vi "Assign Pixel to Wing Sector (FPGA).vi"(6 "Pixel Intensity In":u8, 7 "Right Wing?":bool, 8 "Sector Parameters":T1, 9 "Pixel Y":u16, 10 "Pixel X":u16) -> (1 "Pixel Intensity Out":u8, 2 "sector #":u8, 3 "output valid":bool)   [LabVIEW 2013, in "FPGA Image Processing.lvlib"]
uses:
  FPGA Image Processing.lvlib
  Sector/Accumulate/Sector Parameter Cluster.ctl
  <vilib>/rvi/FXPMathLib/FxpRectToPolar/subVIs/nifxpmath_RectToPolar_SimConfig.ctl
  <vilib>/rvi/FXPMathLib/FxpDiv/subVIs/nifxpmath_Div_SimConfig.ctl
  <vilib>/rvi/FXPMathLib/FxpRectToPolar/simVIs/DllFxpRectToPolarTemp_sub.vi
  <vilib>/rvi/FXPMathLib/FxpDiv/simVIs/DllFxpDivTemp_sub.vi
  <vilib>/rvi/FXPMathLib/FxpSub/XNode/nifxpmath_Sub.xnode
  <vilib>/rvi/FXPMathLib/FxpRectToPolar/XNode/nifxpmath_RectToPolar.xnode
  <vilib>/rvi/FXPMathLib/FxpAdd/XNode/nifxpmath_Add.xnode
  <vilib>/rvi/FXPMathLib/FxpDiv/XNode/nifxpmath_Div.xnode
  <vilib>/rvi/FXPMathLib/sim/FxpSim.dll
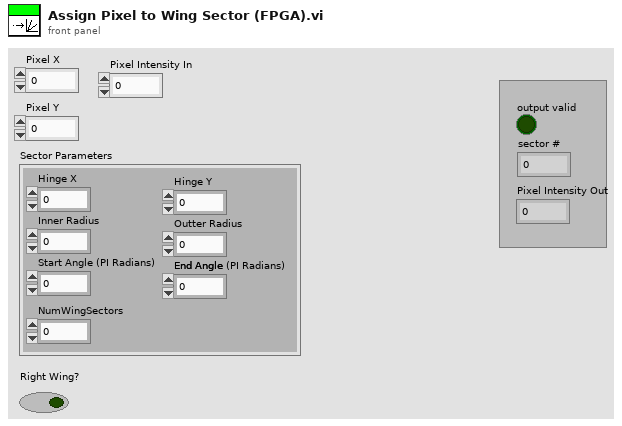
[diagram p1: front panel]
types:
  T1 = typedef "Sector Parameter Cluster.ctl" = cluster{"Start Angle":fxp<+,17,3>, "End Angle":fxp<+,17,3>, "Inner Radius":u16, "Outter Radius":u16, "Hinge X":u16, "Hinge Y":u16, "NumWingSectors":u8}
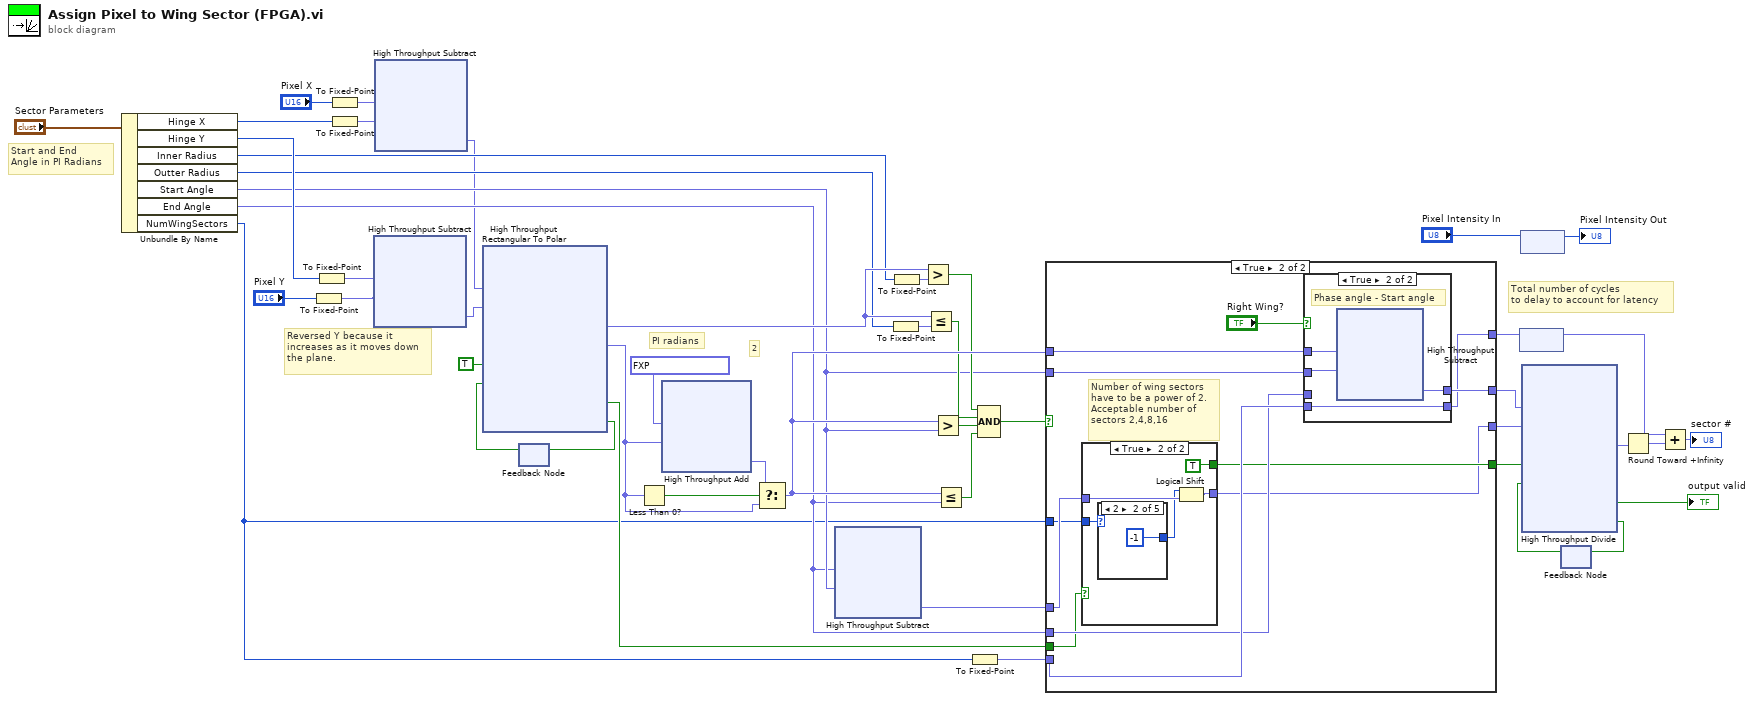
[diagram p0: block diagram]
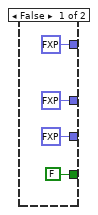
[diagram p2: hidden frame]
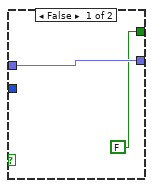
[diagram p3: hidden frame]
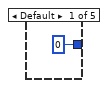
[diagram p4: hidden frame]
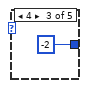
[diagram p5: hidden frame]
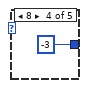
[diagram p6: hidden frame]
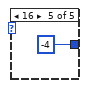
[diagram p7: hidden frame]
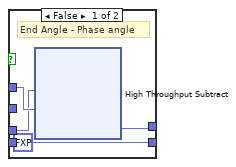
[diagram p8: hidden frame]
diagram:
  # "Reversed Y because it\nincreases as it moves down\nthe plane."
  # "PI radians"
  # "Total number of cycles\nto delay to account for latency"
  # "Start and End\nAngle in PI Radians"
  # "2"
  n1 = Unbundle By Name("Sector Parameters") -> ("Hinge X"=w29:u16, "Hinge Y"=w28:u16, "Inner Radius"=w27:u16, "Outter Radius"=w26:u16, "Start Angle"=w25:fxp<+,17,3>, "End Angle"=w24:fxp<+,17,3>, "NumWingSectors"=w3:u8)
  n2 = To Fixed-Point(number="Pixel Y") -> (fixed-point=w8:fxp<+,11,11>)  [unwired: 1 in]
  n3 = To Fixed-Point(number=w28) -> (fixed-point=w9:fxp<+,11,11>)  [unwired: 1 in]
  n4 = To Fixed-Point(number="Pixel X") -> (fixed-point=w7:fxp<+,11,11>)  [unwired: 1 in]
  n5 = To Fixed-Point(number=w29) -> (fixed-point=w6:fxp<+,11,11>)  [unwired: 1 in]
  n6 = xnode "High Throughput Subtract"("x"=w9, "y"=w8) -> ("x-y"=w22:fxp<+/-,12,12>)
  n7 = xnode "High Throughput Subtract"("x"=w7, "y"=w6) -> ("x-y"=w21:fxp<+/-,12,12>)
  n8 = feedback #1() -> (w37:bool)  [unwired: 1 in]
  n9 = xnode "High Throughput Rectangular To Polar"("x"=w21, "y"=w22, "input valid"=TRUE, "ready for output (T)"=w37) -> ("magnitude"=w47:fxp<+,12,12>, "phase (pi)"=w43:fxp<+/-,16,2>, "output valid"=w4:bool, "ready for input"=w38:bool)
  n10 = feedback-in #1(w38) -> ()
  n11 = Less Than 0?(x=w43) -> (x < 0?=w44:bool)
  n12 = xnode ("High Throughput Add")("x"=fxp<+/-,16,2> 1.99993896484375 ("y"), "y"=w43) -> ("x+y"=w42:fxp<+/-,17,3>)
  n13 = Select(t=w42, s=w44, f=w43) -> (s? t:f=w40:fxp<+/-,17,3>)
  n14 = xnode ("High Throughput Subtract")("x"=w24, "y"=w25) -> ("x-y"=w5:fxp<+/-,17,6>)
  n15 = To Fixed-Point(number=w26) -> (fixed-point=w46:fxp<+,16,16>)  [unwired: 1 in]
  n16 = To Fixed-Point(number=w27) -> (fixed-point=w48:fxp<+,16,16>)  [unwired: 1 in]
  n17 = Greater?(x=w47, y=w48) -> (0:w34:bool)
  n18 = Less Or Equal?(x=w47, y=w46) -> (x <= y?=w33:bool)
  n19 = Greater?(x=w40, y=w25) -> (0:w32:bool)
  n20 = Less Or Equal?(x=w40, y=w24) -> (x <= y?=w31:bool)
  n21 = To Fixed-Point(number=w3) -> (fixed-point=w23:fxp<+,8,8>)  [unwired: 1 in]
  n22 = Compound Arithmetic op=AND(w34, w33, w32, w31) -> (w45:bool)
  n23 = case shown="True" w45 {
    tunnel: w40 -> [_ w64]
    tunnel: w25 -> [_ w63]
    tunnel: [fxp<+/-,17,6> 0.0 ("x-y") w53] -> w16
    tunnel: w24 -> [_ w60]
    tunnel: w23 -> [_ w61]
    tunnel: [fxp<+/-,19,5> 0.0 ("x-y") w59] -> w17
    tunnel: [FALSE ("output valid") w54] -> w15
    tunnel: [fxp<+,8,8> 0.0 w58] -> w12
    tunnel: w5 -> [_ w57]
    tunnel: w4 -> [_ w56]
    tunnel: w3 -> [_ w55]
    frame False {
    }
    frame True {
      # "Number of wing sectors\nhave to be a power of 2.\nAcceptable number of\nsectors 2,4,8,16"
      n24 = case shown="True" w56 {
        tunnel: w55 -> [_ w71]
        tunnel: w57 -> [w66 w70]
        tunnel: [w66 w68] -> w53
        tunnel: [FALSE ("output valid") TRUE ("output valid")] -> w54
        frame False {
        }
        frame True {
          n25 = case shown="2" w71 {
            tunnel: [i16 0 ("y") i16 -1 ("y") i16 -2 ("y") i16 -3 ("y") i16 -4 ("y")] -> w69
            frame Default {
            }
            frame 2 {
            }
            frame 4 {
            }
            frame 8 {
            }
            frame 16 {
            }
          }
          n26 = Logical Shift(y=w69, x=w70) -> (x << y=w68:fxp<+/-,17,6>)
        }
      }
      n27 = case shown="True" "Right Wing?" {
        tunnel: w64 -> [w79 w84]
        tunnel: w63 -> [_ w83]
        tunnel: [w80 w82] -> w59
        tunnel: w61 -> [_ w81]
        tunnel: [fxp<+,8,8> 0.0 w81] -> w58
        tunnel: w60 -> [w78 _]
        frame False {
          # "End Angle - Phase angle"
          n28 = xnode "High Throughput Subtract"("x"=w78, "y"=w79) -> ("x-y"=w80:fxp<+/-,19,5>)
        }
        frame True {
          # "Phase angle - Start angle"
          n29 = xnode ("High Throughput Subtract")("x"=w84, "y"=w83) -> ("x-y"=w82:fxp<+/-,19,5>)
        }
      }
    }
  }
  n30 = feedback #2() -> (w13:fxp<+,8,8>)  [unwired: 1 in]
  n31 = feedback-in #2(w12) -> ()
  n32 = feedback #3() -> (→"Pixel Intensity Out":u8)  [unwired: 1 in]
  n33 = feedback-in #3("Pixel Intensity In") -> ()
  n34 = feedback #4() -> (w14:bool)  [unwired: 1 in]
  n35 = xnode "High Throughput Divide"("x"=w17, "y"=w16, "input valid"=w15, "ready for output (T)"=w14) -> ("x/y"=w11:fxp<+/-,19,16>, "output valid"=→"output valid":bool, "ready for input"=w20:bool)
  n36 = feedback-in #4(w20) -> ()
  n37 = Round Toward +Infinity(x=w11) -> (ceil(x): smallest int >= x=w10:fxp<+/-,17,17>)
  n38 = Add(x=w13, y=w10) -> (x+y=→"sector #":fxp<+/-,17,17>)
